vi "ZoneShift.vi"(10 "LineDir":bool) -> ()   [LabVIEW 2013]
uses:
  Robot Global Data.vi
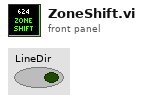
[diagram p1: front panel]
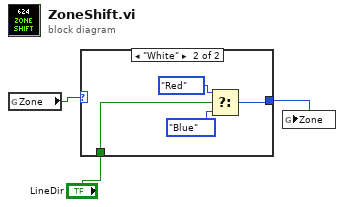
[diagram p0: block diagram]
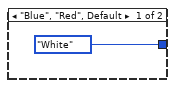
[diagram p2: hidden frame]
diagram:
  n1 = global read "Robot Global Data.vi" "Zone"() -> (w3:enum16{"Blue", "White", "Red"})
  n2 = case shown="\"White\"" w3 {
    tunnel: [enum16{"Blue", "White", "Red"}."White" ("Zone") w8] -> w2
    tunnel: "LineDir" -> [_ w5]
    frame "Blue", "Red", Default {
    }
    frame "White" {
      n3 = Select(t=enum16{"Blue", "White", "Red"}."Red" ("Zone"), s=w5, f=enum16{"Blue", "White", "Red"}."Blue") -> (s? t:f=w8:enum16{"Blue", "White", "Red"})
    }
  }
  n4 = global write "Robot Global Data.vi" "Zone"(w2) -> ()
